vi "Init.vi"(8 "error in (no error)":errorcluster, 10 "Eye Params":dbl[](array[numeric]), 11 "TrialBasedExperiment in":refnum<class "DotMapping.lvclass">) -> (0 "error out":errorcluster, 3 "TrialBasedExperiment out":refnum<class "DotMapping.lvclass">)   [LabVIEW 2010, in "DotMapping.lvclass"]
uses:
  DotMapping.lvclass
  PassiveExperiment/PassiveExperiment.lvclass
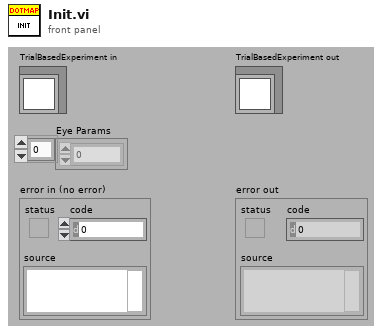
[diagram p1: front panel]
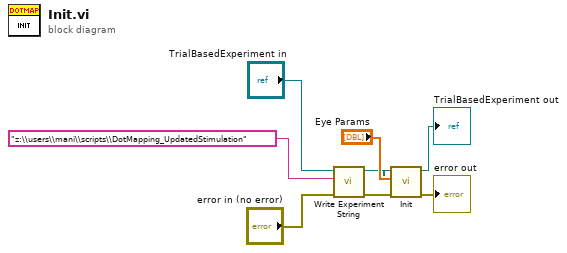
[diagram p0: block diagram]
diagram:
  n1 = call-dynamic "Write Experiment String.vi"("error in (no error)"="error in (no error)", "Experiment String"="z:\\users\\mani\\scripts\\DotMapping_UpdatedStimulation", "TrialBasedExperiment in"="TrialBasedExperiment in") -> ("error out"=w4:errorcluster, "TrialBasedExperiment out"=w2:refnum<class "DotMapping.lvclass">)  [unwired: 7 in]
  n2 = call-parent "Init.vi"("error in (no error)"=w4, "Eye Params"="Eye Params", "TrialBasedExperiment in"=w2) -> ("error out"=→"error out":errorcluster, "TrialBasedExperiment out"=→"TrialBasedExperiment out":refnum<class "DotMapping.lvclass">)  [unwired: 7 in]
